vi "hmi_LM_API_UPD_SEND_DATA.vi"(6 "data":u8[](array[numeric]) format="%.0x", 8 "Error in":errorcluster {"code" format="%.0x"}, 11 "canSession":T1) -> (0 "Error out":errorcluster {"code" format="%.0x"}, 1 "msgData":T2[](array[typedef]) {"Data" format="%.0x"; "ArbitrationId" format="%.0x"; "Timestamp" format="%<%I:%M:%S%3u %p\n%m/%d/%Y>T"}, 3 "canSession":T1)   [LabVIEW 2017]
doc: "Demonstrates how to write and receive CAN frames via the Network Interface on the same port. \n\nTo write and receive frames via the Network Interface:\n- select the CAN Network Interface (i.e. CAN0, CAN1, etc.)\n- select the Baud Rate\n- run the VI\n- press the write button to write frames to the can bus\n\nEnable RTR Button to send a Remote Transmission Request or to simply send an empty Frame to request an Answer Frame from a connected device.\n\nEnable Extended Button to write extended Identifier Format. This is done by setting the 30th bit to enable extended format with the driver."
uses:
  <vilib>/nican/nican.llb/CanFrameTimed.ctl
  <vilib>/nican/nican.llb/xobjhandle.ctl
  LM_API_UPD.ctl
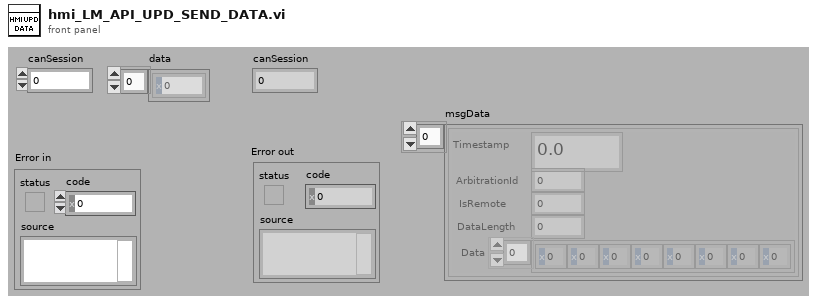
[diagram p1: front panel]
types:
  T1 = typedef "xobjhandle.ctl" = u32
  T2 = typedef "CanFrameTimed.ctl" = cluster{"Timestamp":dbl, "ArbitrationId":u32, "IsRemote":u8, "DataLength":u8, "Data":u8[]}
  T3 = typedef "LM_API_UPD.ctl" = u32
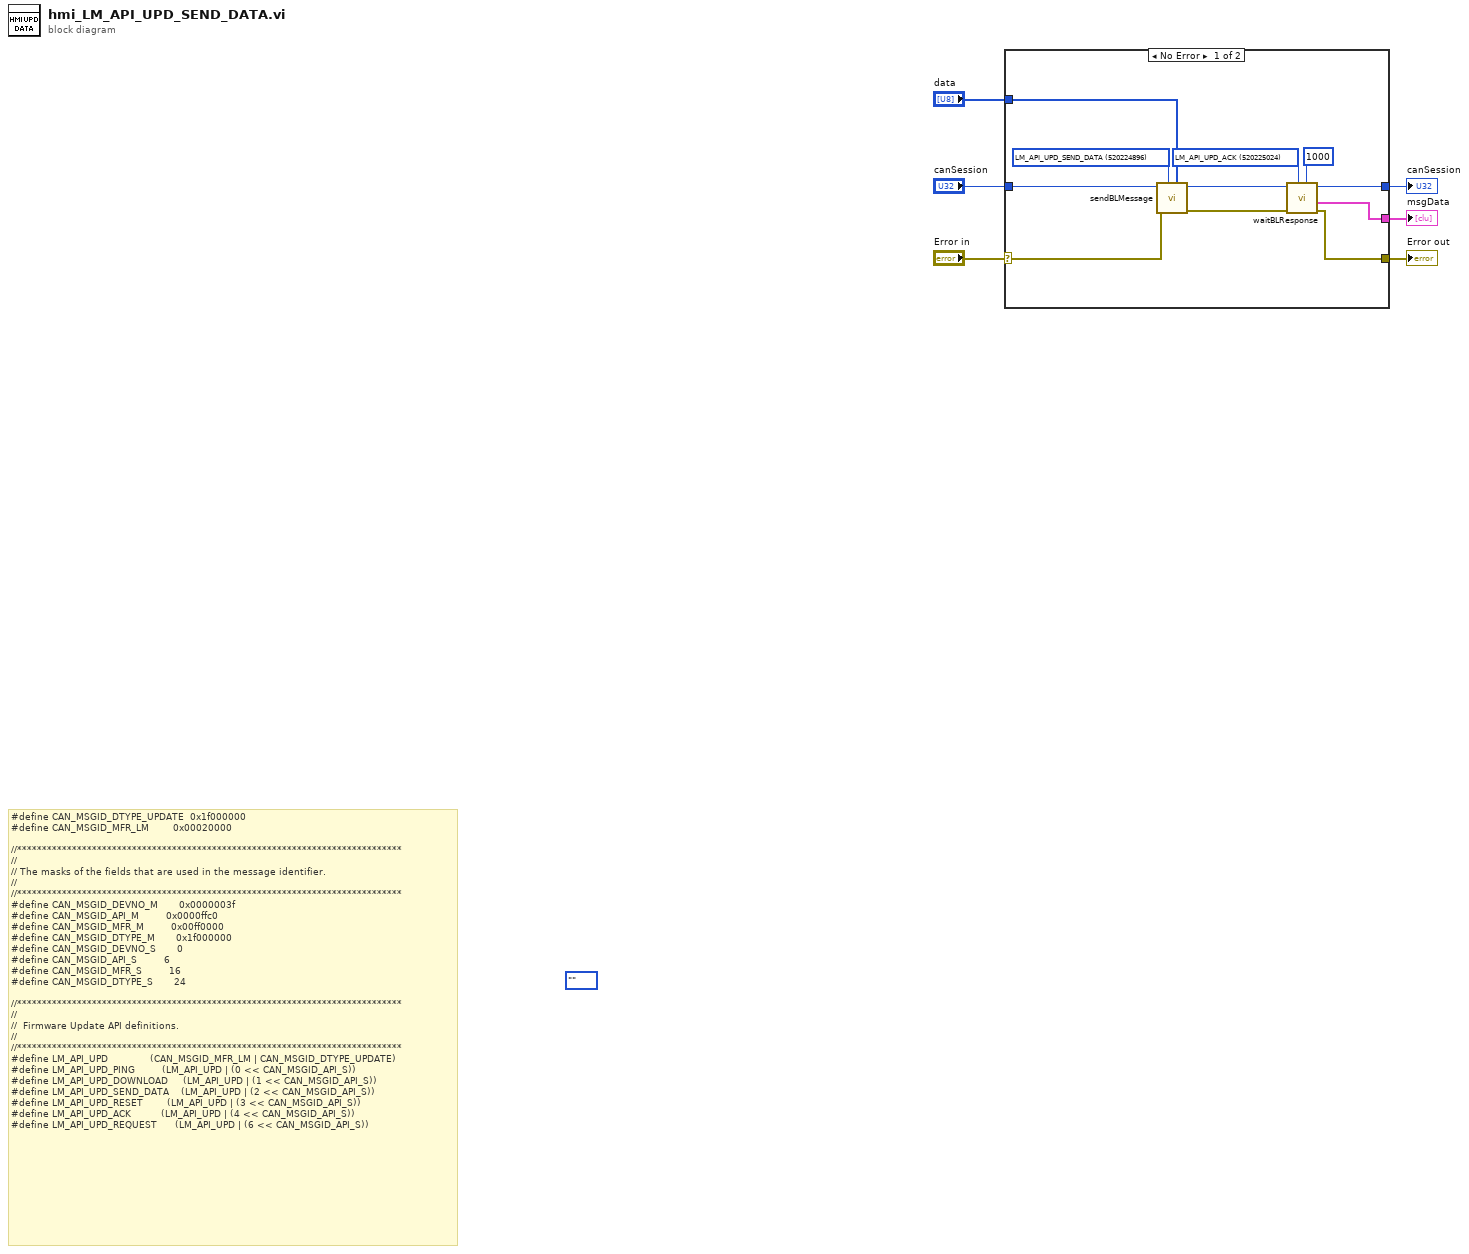
[diagram p0: block diagram]
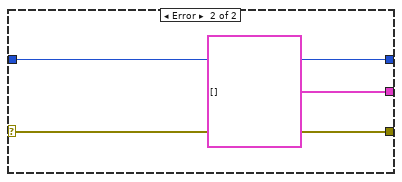
[diagram p2: hidden frame]
diagram:
  (unwired) enum32{""}.""
  # "#define CAN_MSGID_DTYPE_UPDATE  0x1f000000\n#define CAN_MSGID_MFR_LM        0x00020000\n\n//*****************************************************************************\n//\n// The masks of the fields that are used in the message identifier.\n//\n//*****************************************************************************\n#define CAN_MSGID_DEVNO_M       0x0000003f\n#define CAN_MSGID_API_M         0x0000ffc0\n#define CAN_MSGID_MFR_M         0x00ff0000\n#define CAN_MSGID_DTYPE_M       0x1f000000\n#define CAN_MSGID_DEVNO_S       0\n#define CAN_MSGID_API_S         6\n#define CAN_MSGID_MFR_S         16\n#define CAN_MSGID_DTYPE_S       24\n\n//*****************************************************************************\n//\n//  Firmware Update API definitions.\n//\n//*****************************************************************************\n#define LM_API_UPD              (CAN_MSGID_MFR_LM | CAN_MSGID_DTYPE_UPDATE)\n#define LM_API_UPD_PING         (LM_API_UPD | (0 << CAN_MSGID_API_S))\n#define LM_API_UPD_DOWNLOAD     (LM_API_UPD | (1 << CAN_MSGID_API_S))\n#define LM_API_UPD_SEND_DATA    (LM_API_UPD | (2 << CAN_MSGID_API_S))\n#define LM_API_UPD_RESET        (LM_API_UPD | (3 << CAN_MSGID_API_S))\n#define LM_API_UPD_ACK          (LM_API_UPD | (4 << CAN_MSGID_API_S))\n#define LM_API_UPD_REQUEST      (LM_API_UPD | (6 << CAN_MSGID_API_S))"
  n1 = case shown="No Error" "Error in" {
    selector: "Error in" -> [w10 w20]
    tunnel: [w15 T2[] [] ("msgData")] -> w6
    tunnel: "canSession" -> [w14 w19]
    tunnel: [w13 w19] -> w4
    tunnel: [w12 w20] -> w3
    tunnel: "data" -> [w7 _]
    frame No Error {
      w8 = T3 520224896 items=["LM_API_UPD_PING"=520224768, "LM_API_UPD_DOWNLOAD"=520224832, "LM_API_UPD_SEND_DATA"=520224896, "LM_API_UPD_RESET"=520224960, "LM_API_UPD_ACK"=520225024, "LM_API_UPD_REQUEST"=520225152] ("Response")
      w9 = T3 520225024 items=["LM_API_UPD_PING"=520224768, "LM_API_UPD_DOWNLOAD"=520224832, "LM_API_UPD_SEND_DATA"=520224896, "LM_API_UPD_RESET"=520224960, "LM_API_UPD_ACK"=520225024, "LM_API_UPD_REQUEST"=520225152] ("Response")
      n2 = call "sendBLMessage.vi"("blMessageData"=w7, "blMessage"=w8, "Error in"=w10, "ObjHandle in"=w14) -> ("Error out"=w16:errorcluster, "ObjHandle out"=w17:T1)  [unwired: 6 in]
      n3 = call "waitBLResponse.vi"("timout(ms)"=u32 1000, "Response"=w9, "Error in"=w16, "ObjHandle in"=w17) -> ("Error out"=w12:errorcluster, "msgData"=w15:T2[], "ObjHandle out"=w13:T1)  [unwired: 4 in, 1 out]
    }
    frame Error {
    }
  }
  "msgData" <- w6
  "canSession" <- w4
  "Error out" <- w3
